vi "Configure Display.vi"(0 "VISA resource name":refnum<visa-resource-name>, 1 "Display Brightness (2:75%)":u16(ring)=2 items=["25%", "50%", "75%", "100%"], 5 "Display Mode (0:Input A)":u16(ring) items=["Input A", "Input A Max/Min", "Two Input, Loop A", "Input B", "Input B Max/Min", "Two Input, Loop B", "Custom", "Two Loop"], 7 "Front Panel LEDs (T: On)":bool=TRUE, 11 "error in (no error)":errorcluster, 12 "Field to Configure (1)":dbl=1.0, 13 "Input (0:None)":u16(ring) items=["None", "Input A", "Input B", "Setpoint 1", "Setpoint 2", "Output 1", "Output 2"], 14 "Units (1:Kelvin)":u16(ring)=1 items=["Kelvin"=1, "Celsius"=2, "Sensor Units"=3, "Minimum Data"=4, "Maximum Data"=5, "Sensor Name"=6]) -> (4 "VISA resource name out":refnum<visa-resource-name>, 15 "error out":errorcluster)   [LabVIEW 2012, in "Lake Shore 335.lvlib"]
doc: "Configures the Model 335 front panel display settings. The Model 335 provides four display modes designed to accommodate different instrument configurations and user preferences. The display modes are listed here.\n\n<B>Two Input One Loop Display Mode</B> \nProvides both sensor readings, as well as control loop information for one control loop.\n\n<B>Two Loop Display Mode</B>\nProvides the sensor reading and control setpoint for both control loops.\n\n<B>Input Display Mode</B>\nProvides detailed information about the relevant sensor input, and the associated output.\n\n<B>Custom Display Mode</B>\nProvides a means for you to assign different types of information to specific sections of the display."
uses:
  <instrlib>/lake shore 335/Temperature control panel Folder/C/Program Files/National Instruments/LabVIEW 2013/instr.lib/lake shore 335/Lake Shore 335.lvlib
  Instance           1 25Saved   Configure Display .vi
panel:
  # "Custom Display Mode Settings"
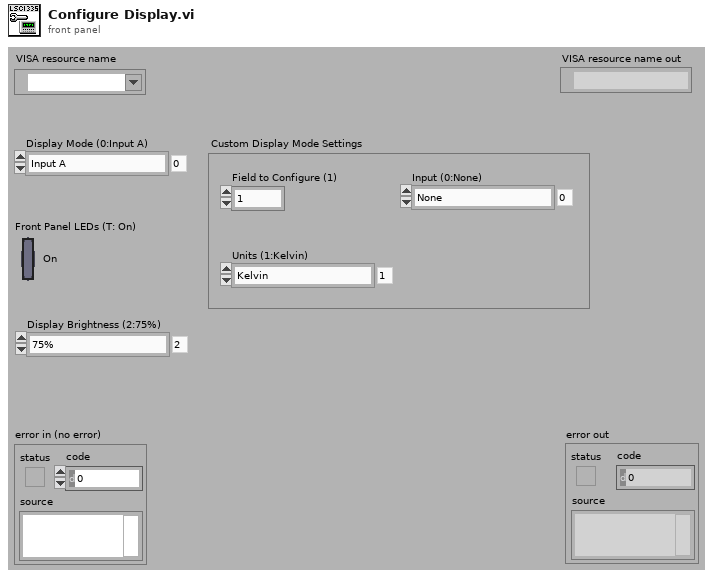
[diagram p1: front panel]
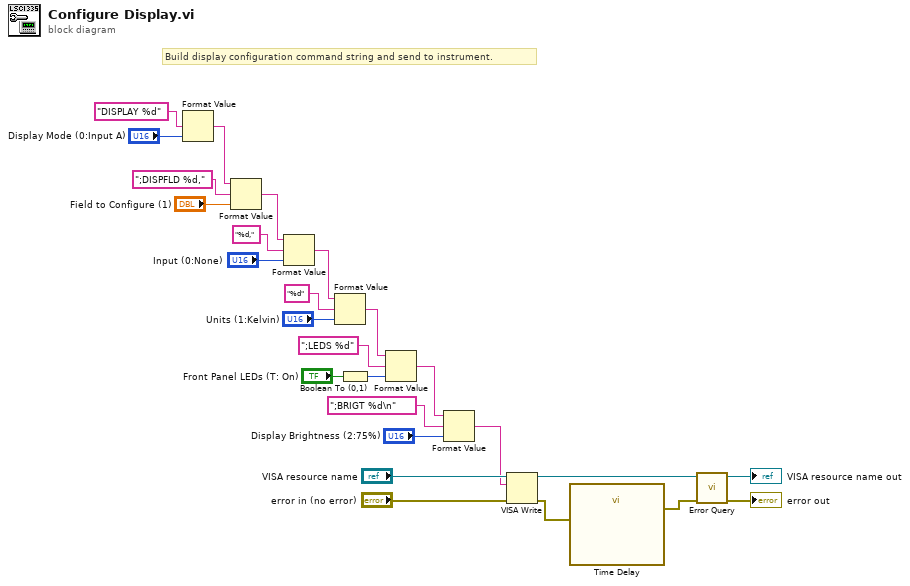
[diagram p0: block diagram]
diagram:
  # "Build display configuration command string and send to instrument."
  n1 = Format Value(format string="DISPLAY %d", value (0)="Display Mode (0:Input A)") -> (output string=w2:string)  [unwired: 1 in]
  n2 = Format Value(string ("")=w2, format string=";DISPFLD %d,", value (0)="Field to Configure (1)") -> (output string=w17:string)
  n3 = Format Value(string ("")=w17, format string="%d,", value (0)="Input (0:None)") -> (output string=w15:string)
  n4 = Format Value(string ("")=w15, format string="%d", value (0)="Units (1:Kelvin)") -> (output string=w6:string)
  n5 = Boolean To (0,1)(Boolean="Front Panel LEDs (T: On)") -> (0, 1=w9:i16)
  n6 = Format Value(string ("")=w6, format string=";LEDS %d", value (0)=w9) -> (output string=w4:string)
  n7 = Format Value(string ("")=w4, format string=";BRIGT %d\n", value (0)="Display Brightness (2:75%)") -> (output string=w3:string)
  n8 = VISA Write(VISA resource name="VISA resource name", write buffer=w3, error in (no error)="error in (no error)") -> (VISA resource name out=w23:refnum<visa-resource-name>, error out=w13:errorcluster)  [unwired: 1 out]
  n9 = call "Time Delay"("error in (no error)"=w13) -> ("error out"=w12:errorcluster)  [unwired: 10 in]
  n10 = call <instrlib>:"Error Query.vi"("error in (no error)"=w12, "VISA resource name"=w23) -> ("error out"=→"error out":errorcluster, "VISA resource name out"=→"VISA resource name out":refnum<visa-resource-name>)  [unwired: 7 in, 1 out]
